vi "ZSlice compute-core_old-ref.vi"(11 "ZStack (um)":cluster{"Zstart":dbl, "Zstop":dbl, "Zstep":dbl}) -> (1 "Motor Z Planes(um)":dbl[](array[numeric]) format="%#_12f", 2 "# of Z-planes":i32, 3 "AOL Z Planes(um)":dbl[](array[numeric]) format="%#_12f")   [LabVIEW 2020]
uses:
  Global Variables/General Globals.vi
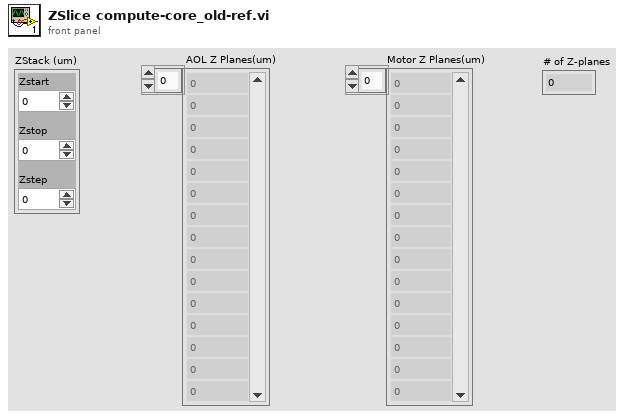
[diagram p1: front panel]
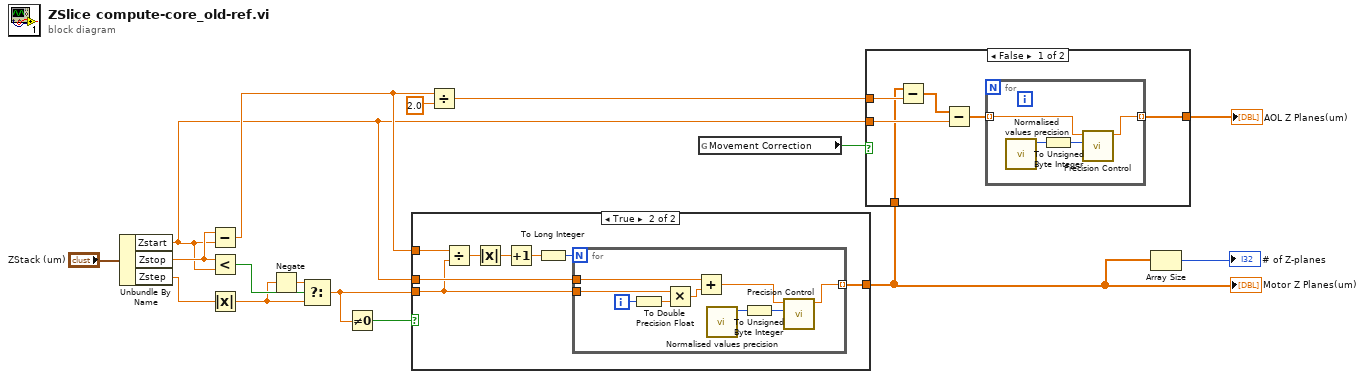
[diagram p0: block diagram]
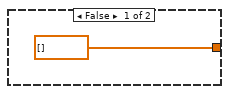
[diagram p3: hidden frame]
diagram:
  n1 = Unbundle By Name("ZStack (um)") -> ("Zstart"=w6:dbl, "Zstop"=w13:dbl, "Zstep"=w12:dbl)
  n2 = Subtract(x=w13, y=w6) -> (x-y=w9:dbl)
  n3 = Less?(x=w13, y=w6) -> (x < y?=w16:bool)
  n4 = Absolute Value(x=w12) -> (abs(x)=w14:dbl)
  n5 = Negate(x=w14) -> (-x=w15:dbl)
  n6 = Select(t=w15, s=w16, f=w14) -> (s? t:f=w11:dbl)
  n7 = Not Equal To 0?(x=w11) -> (x != 0?=w10:bool)
  n8 = case shown="True" w10 {
    tunnel: w9 -> [_ w25]
    tunnel: w6 -> [_ w21]
    tunnel: w11 -> [_ w20]
    tunnel: [dbl[] [] w19] -> w2
    frame False {
    }
    frame True {
      n9 = Divide(x=w25, y=w20) -> (x/y=w22:dbl)
      n10 = Absolute Value(x=w22) -> (abs(x)=w23:dbl)
      n11 = Increment(x=w23) -> (x+1=w24:dbl)
      n12 = To Long Integer(number=w24) -> (32bit integer=w18:i32)
      n13 = for {
        N: w18 -> [_]
        tunnel: w20 -> [w33]
        tunnel: w21 -> [w32]
        tunnel: [w26] -> w19 mode=indexing
        i -> [w34]
        n14 = To Double Precision Float(number=w34) -> (double precision float=w30:dbl)
        n15 = Multiply(x=w33, y=w30) -> (x*y=w31:dbl)
        n16 = Add(x=w32, y=w31) -> (x+y=w27:dbl)
        n17 = call "Normalised values precision.vi"() -> ("Normalised values precision"=w28:i32)  [unwired: 11 in]
        n18 = To Unsigned Byte Integer(number=w28) -> (unsigned 8bit integer=w29:u8)
        n19 = call <userlib>:"Precision Control.vi"("Precision"=w29, "Input Value"=w27) -> ("Output Value"=w26:dbl)  [unwired: 8 in, 1 out]
      }
    }
  }
  "Motor Z Planes(um)" <- w2
  n20 = Divide(x=w9, y=2.0) -> (x/y=w7:dbl)
  n21 = global read "General Globals.vi" "Movement Correction"() -> (w1:bool)
  n22 = case shown="False" w1 {
    tunnel: w7 -> [w39 _]
    tunnel: w6 -> [w38 _]
    tunnel: [w36 w45] -> w4
    tunnel: w2 -> [w35 w45]
    frame False {
      n23 = Subtract(x=w35, y=w39) -> (x-y=w40:dbl[])
      n24 = Subtract(x=w40, y=w38) -> (x-y=w37:dbl[])
      n25 = for {
        tunnel: [w42] -> w36 mode=indexing
        tunnel: w37 -> [w41] mode=indexing
        n26 = call "Normalised values precision.vi"() -> ("Normalised values precision"=w43:i32)  [unwired: 11 in]
        n27 = To Unsigned Byte Integer(number=w43) -> (unsigned 8bit integer=w44:u8)
        n28 = call <userlib>:"Precision Control.vi"("Precision"=w44, "Input Value"=w41) -> ("Output Value"=w42:dbl)  [unwired: 8 in, 1 out]
      }
    }
    frame True {
    }
  }
  "AOL Z Planes(um)" <- w4
  n29 = Array Size(array=w2) -> (size(s)=→"# of Z-planes":i32)
